vi "AG Spreadsheet.vi"() -> ()   [LabVIEW 2012]
uses:
  Controls/Spreadsheet_Messege.ctl
  <vilib>/Utility/sysdir.llb/System Directory Type.ctl
  Controls/Spreadsheet Commands.ctl
  Utilities/AG Tab Action.ctl
  Controls/Sheet Colors.ctl
  ActivityGuideEvents.ctl
panel:
  in  "Clear Sheet":bool
  in  "Copy to Clipboard":bool
  in  "Save as .csv":bool
  in  "Blank Button":bool
  in  "Sheet Colors":T1={"Header Color"=16711680, "Header Font Color"=16448250, "Font Color"=0, "Clear Color"=16448250, "Alt Clear Color"=13224393}
  in  "Resources":path[](array[path])
  in  "TabButtonsRef":refnum<vi>
  in  "Multicolumn Listbox":i32[](listbox)
  in  "ActivityGuideEvents":T2
  # "Spreadsheet Title"
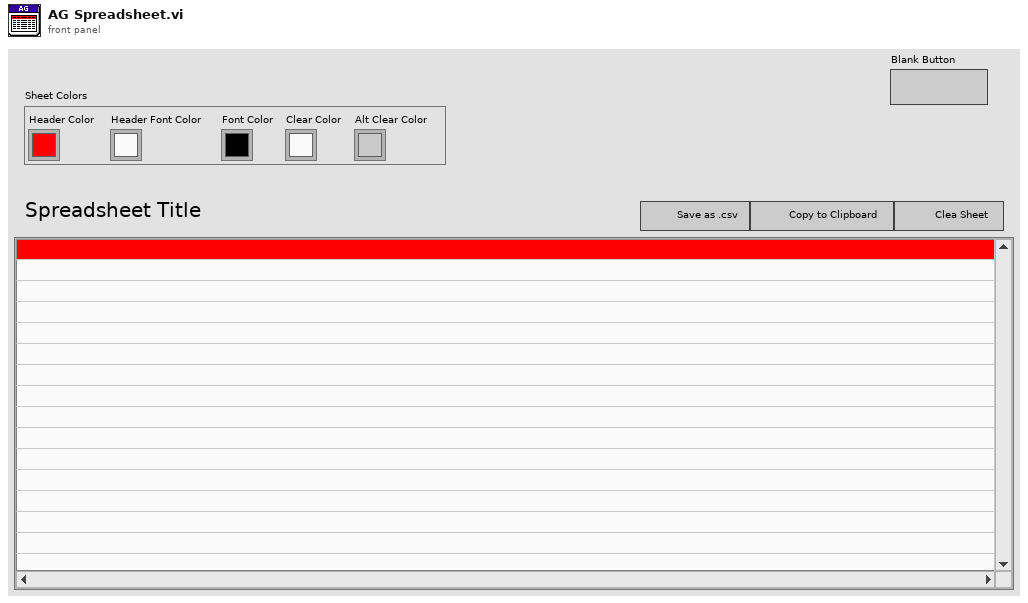
[diagram p1: front panel]
types:
  T1 = typedef "Sheet Colors.ctl" = cluster{"Header Color":u32, "Header Font Color":u32, "Font Color":u32, "Clear Color":u32, "Alt Clear Color":u32}
  T2 = typedef "ActivityGuideEvents.ctl" = refnum<event-registration>
  T3 = typedef "AG Tab Action.ctl" = enum16{"Initilize", "Select", "Blink", "Disable", "KeyFocus", "Set Description", "Hide", "NULL"}
  T4 = typedef "Spreadsheet Commands.ctl" = enum16{"Init", "Clear", "Add", "Mass Add", "Delete Row", "Format Colors"}
  T5 = typedef "Spreadsheet_Messege.ctl" = cluster{"Action (add)":T4, "Data":string[], "2D Data":string[][]}
  T6 = typedef "System Directory Type.ctl" = i32
  T7 = typedef "LVPoint32TypeDef.ctl" = cluster{"Horizontal":i32, "Vertical":i32}
  T8 = typedef "LVRowAndColumnTypeDef.ctl" = cluster{"Row":i32, "Column":i32}
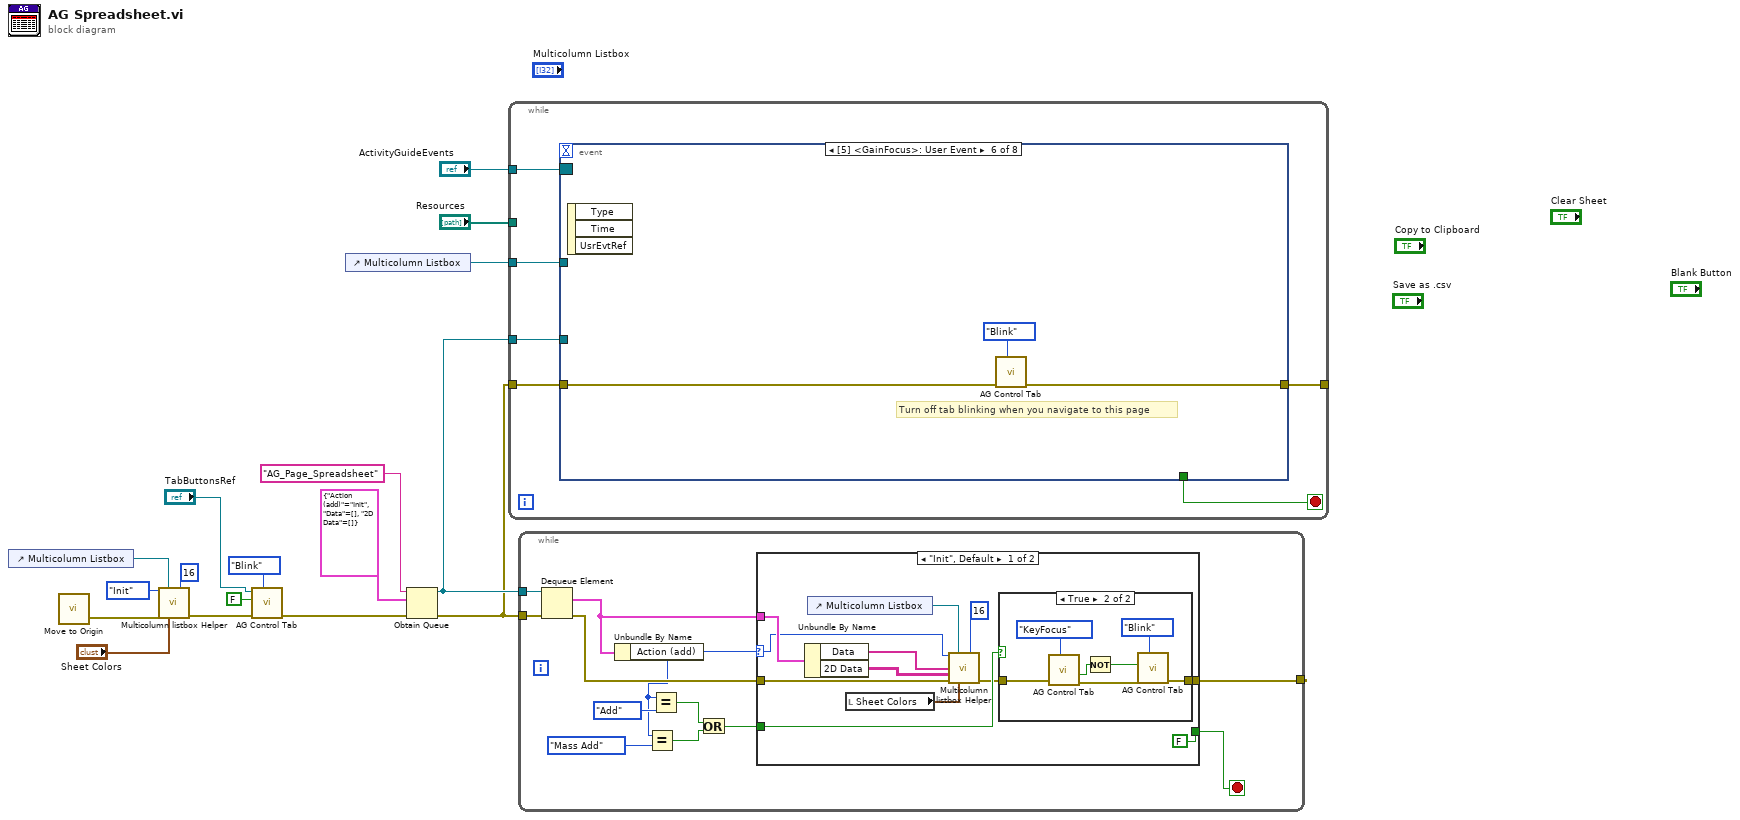
[diagram p0: block diagram]
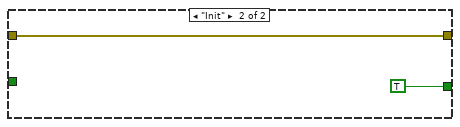
[diagram p3: hidden frame]
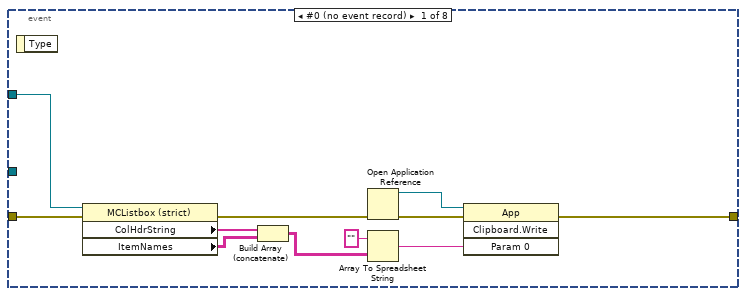
[diagram p4: hidden frame]
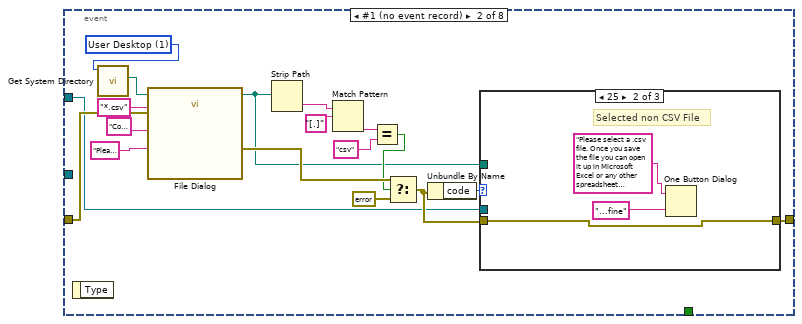
[diagram p5: hidden frame]
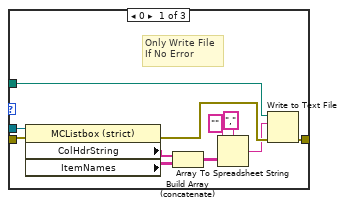
[diagram p6: hidden frame]
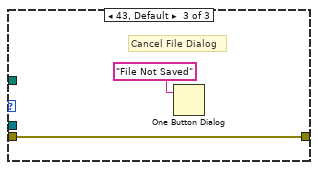
[diagram p7: hidden frame]
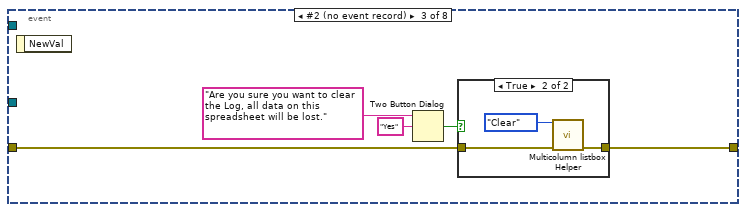
[diagram p8: hidden frame]
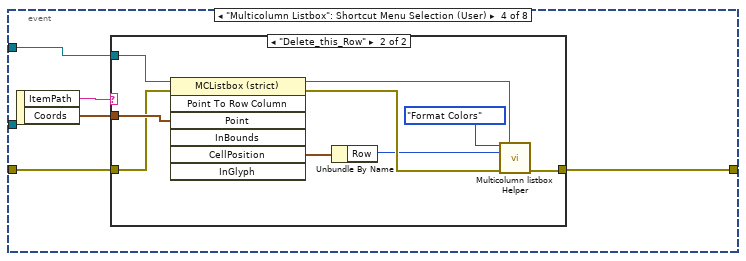
[diagram p10: hidden frame]
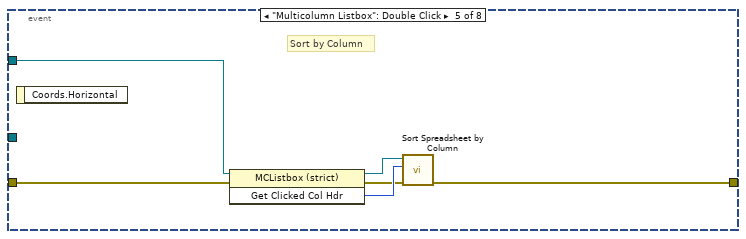
[diagram p12: hidden frame]
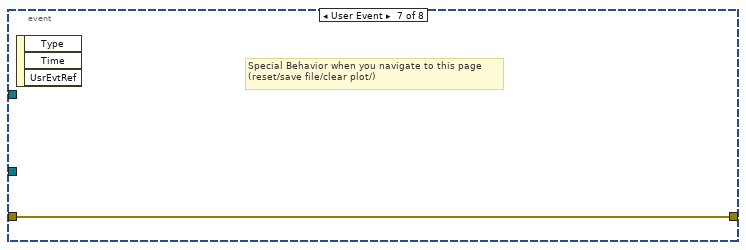
[diagram p13: hidden frame]
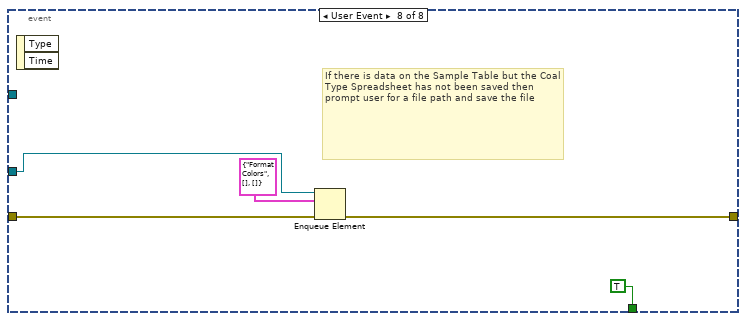
[diagram p14: hidden frame]
diagram:
  n1 = control-ref of="Multicolumn Listbox"() -> (w11:refnum<vi>)
  n2 = call "Move to Origin.vi"() -> ("Error Out"=w2:errorcluster)  [unwired: 3 in]
  n3 = call "Multicolumn listbox Helper.vi"("Action (add default)"=Spreadsheet_Commands."Init", "Multicolumn Ref"=w11, "Visible rows"=16, "Error In"=w2, "Sheet Colors"="Sheet Colors") -> ("Error Out"=w7:errorcluster)  [unwired: 10 in]
  n4 = call "AG Control Tab.vi"("Action (Init)"=AG_Tab_Action."Blink" ("Action"), "error in (no error)"=w7, "Value(F)"=FALSE, "TabButtonsRef"="TabButtonsRef") -> ("error out"=w1:errorcluster)  [unwired: 4 in, 3 out]
  n5 = control-ref of="Multicolumn Listbox"() -> (w13:refnum<vi>)
  n6 = Obtain Queue(name (unnamed)="AG_Page_Spreadsheet", element data type=T5 {"Action (add)"=enum."Init", "Data"=[], "2D Data"=[]} ("Cluster"), error in (no error)=w1) -> (queue out=w14:refnum<queue>, error out=w10:errorcluster)  [unwired: 2 in, 1 out]
  n7 = while {
    tunnel: "ActivityGuideEvents" -> [w23]
    tunnel: w14 -> [w21]
    tunnel: w13 -> [w20]
    tunnel: [w19] -> _
    tunnel: w10 -> [w18]
    tunnel: "Resources" -> [_]
    stop <- w22 stop-if-true
    n8 = event shown="[5] <GainFocus>: User Event" {
      selector: w23 -> [_ _ _ _ _ _ _ _]
      dyn-events: _ -> [_ _ _ _ _ _ _ _]
      timeout: _ -> [_ _ _ _ _ _ _ _]
      tunnel: [_ _ _ _ _ _ _ TRUE] -> w22
      tunnel: w21 -> [_ _ _ _ _ _ _ w103]
      tunnel: w20 -> [w31 w35 _ w78 w95 _ _ _]
      tunnel: [w27 w38 w70 w81 w94 w100 w102 w105] -> w19
      tunnel: w18 -> [w25 w36 w69 w80 w93 w99 w102 w104]
      event #0 (no event record) {
        n9 = event-data() -> ()  [unwired: 1 in, 1 out]
        n10 = property class="MCListbox (strict)"(reference=w31, error in=w25) -> (error out=w26:errorcluster, "ColHdrString"=w30:string[], "ItemNames"=w29:string[][])  [unwired: 1 out]
        n11 = Build Array (concatenate)(w30, w29) -> (w28:string[][])
        n12 = Open Application Reference(8:w26) -> (0:w32:errorcluster, 3:w24:refnum<vi>)  [unwired: 3 in]
        n13 = Array To Spreadsheet String(array=w28, 3:"" ("format string")) -> (spreadsheet string=w33:string)  [unwired: 1 in]
        n14 = invoke class="App" method="Clipboard.Write"(reference=w24, error in=w32, "Param 0"=w33) -> (error out=w27:errorcluster)  [unwired: 1 in, 3 out]
      }
      event #1 (no event record) {
        w50 = T6 1 items=["User Home"=0, "User Desktop"=1, "User Documents"=2, "User Application Data"=3, "User Preferences"=4, "User Temporary"=5, "Public Documents"=6, "Public Application Data"=7, "Public Preferences"=8, "Public Cache"=13, "System Core Libraries"=9, "System Installed Libraries"=10, "Application Files"=11, "Boot Volume Root"=12] ("system directory type")
        n15 = event-data() -> ()  [unwired: 1 in, 1 out]
        n16 = call <vilib>:"Get System Directory.vi"("system directory type"=w50) -> ("system directory"=w49:path)  [unwired: 10 in]
        n17 = call "File Dialog"("start path"=w49, "prompt"="Please select a file to save your data.", "error in"=w36, "pattern (all files)"="*.csv", "pattern label"="Comma Seperated Value Files") -> ("selected path"=w39:path, "error out"=w42:errorcluster)  [unwired: 7 in, 2 out]
        n18 = Strip Path(path=w39) -> (name=w46:string)  [unwired: 1 out]
        n19 = Match Pattern(string=w46, regular expression="[.]") -> (after substring=w45:string)  [unwired: 1 in, 3 out]
        n20 = Equal?(x=w45, y="csv") -> (x = y?=w40:bool)
        n21 = Select(t=w42, s=w40, f=errorcluster {"status"=TRUE, "code"=25, "source"=""}) -> (s? t:f=w37:errorcluster)
        n22 = Unbundle By Name(w37) -> ("code"=w43:i32)
        n23 = case shown="25" w43 {
          tunnel: w39 -> [w63 _ _]
          tunnel: [w62 w64 w67] -> w38
          tunnel: w37 -> [w55 w64 w67]
          tunnel: w35 -> [w54 _ _]
          frame 0 {
            # "Only Write File\nIf No Error"
            n24 = property class="MCListbox (strict)"(reference=w54, error in=w55) -> (error out=w56:errorcluster, "ColHdrString"=w57:string[], "ItemNames"=w58:string[][])  [unwired: 1 out]
            n25 = Build Array (concatenate)(w57, w58) -> (w59:string[][])
            n26 = Array To Spreadsheet String(delimiter (Tab)=",", array=w59, 3:"" ("format string")) -> (spreadsheet string=w53:string)
            n27 = Write to Text File(file (use dialog)=w63, text=w53, error in=w56) -> (error out=w62:errorcluster)  [unwired: 1 in, 2 out]
          }
          frame 25 {
            # "Selected non CSV File"
            n28 = One Button Dialog(message="Please select a .csv file. Once you save the file you can open it up in Microsoft Excel or any other spreadsheet application. ", button name ("OK")="...fine" ("format string")) -> ()  [unwired: 1 out]
          }
          frame 43, Default {
            # "Cancel File Dialog"
            n29 = One Button Dialog(message="File Not Saved") -> ()  [unwired: 1 in, 1 out]
          }
        }
      }
      event #2 (no event record) {
        n30 = event-data() -> ()  [unwired: 1 in, 1 out]
        n31 = Two Button Dialog(message="Are you sure you want to clear the Log, all data on this spreadsheet will be lost.", 2:"Yes" ("T button name (\"OK\")")) -> (T button?=w71:bool)  [unwired: 1 in]
        n32 = case shown="True" w71 {
          tunnel: [w74 w77] -> w70
          tunnel: w69 -> [w74 w76]
          frame False {
          }
          frame True {
            n33 = call "Multicolumn listbox Helper.vi"("Action (add default)"=Spreadsheet_Commands."Clear", "Error In"=w76) -> ("Error Out"=w77:errorcluster)  [unwired: 13 in]
          }
        }
      }
      event "Multicolumn Listbox": Shortcut Menu Selection (User) {
        n34 = event-data() -> ("ItemPath"=w82:string, "Coords"=w79:T7)  [unwired: 1 in]
        n35 = case shown="\"Delete_this_Row\"" w82 {
          tunnel: [w83 w87] -> w81
          tunnel: w80 -> [w83 w90]
          tunnel: w79 -> [_ w92]
          tunnel: w78 -> [_ w84]
          frame "NULL", Default {
          }
          frame "Delete_this_Row" {
            n36 = invoke class="MCListbox (strict)" method="Point To Row Column"(reference=w84, error in=w90, "Point"=w92) -> (reference out=w89:refnum<vi>, error out=w88:errorcluster, "CellPosition"=w91:T8)  [unwired: 4 in, 4 out]
            n37 = Unbundle By Name(w91) -> ("Row"=w85:i32)
            n38 = call "Multicolumn listbox Helper.vi"("Action (add default)"=Spreadsheet_Commands."Format Colors", "Multicolumn Ref"=w89, "Row to Delete"=w85, "Error In"=w88) -> ("Error Out"=w87:errorcluster)  [unwired: 11 in]
          }
        }
      }
      event "Multicolumn Listbox": Double Click {
        # "Sort by Column"
        n39 = event-data() -> ()  [unwired: 1 in, 1 out]
        n40 = invoke class="MCListbox (strict)" method="Get Clicked Col Hdr"(reference=w95, error in=w93) -> (reference out=w97:refnum<vi>, error out=w96:errorcluster, "Get Clicked Column Header"=w98:i32)  [unwired: 1 in]
        n41 = call "Sort Spreadsheet by Column.vi"("error in (no error)"=w96, "Column Number"=w98, "Ref In"=w97) -> ("error out"=w94:errorcluster)  [unwired: 8 in]
      }
      event User Event {
        # "Turn off tab blinking when you navigate to this page"
        n42 = event-data() -> ()  [unwired: 1 in, 3 out]
        n43 = call "AG Control Tab.vi"("Action (Init)"=AG_Tab_Action."Blink" ("Action"), "error in (no error)"=w99) -> ("error out"=w100:errorcluster)  [unwired: 6 in, 3 out]
      }
      event User Event {
        # "Special Behavior when you navigate to this page\n(reset/save file/clear plot/)"
        n44 = event-data() -> ()  [unwired: 1 in, 3 out]
      }
      event User Event {
        # "If there is data on the Sample Table but the Coal Type Spreadsheet has not been saved then prompt user for a file path and save the file"
        n45 = event-data() -> ()  [unwired: 1 in, 2 out]
        n46 = Enqueue Element(queue=w103, element=T5 {"Action (add)"=enum."Format Colors", "Data"=[], "2D Data"=[]}, error in (no error)=w104) -> (error out=w105:errorcluster)  [unwired: 1 in, 2 out]
      }
    }
  }
  n47 = while {
    tunnel: w14 -> [w119]
    tunnel: w10 -> [w118]
    tunnel: [w108] -> _
    stop <- w117 stop-if-true
    n48 = Dequeue Element(queue=w119, error in (no error)=w118) -> (element=w115:T5, error out=w116:errorcluster)  [unwired: 1 in, 2 out]
    n49 = Unbundle By Name(w115) -> ("Action (add)"=w110:T4)
    n50 = Equal?(x=w110, y=Spreadsheet_Commands."Mass Add" ("Action (add)")) -> (x = y?=w113:bool)
    n51 = Equal?(x=w110, y=Spreadsheet_Commands."Add" ("Action (add)")) -> (x = y?=w114:bool)
    n52 = Or(x=w114, y=w113) -> (x .or. y?=w109:bool)
    n53 = case shown="\"Init\", Default" w110 {
      selector: w110 -> [w125 _]
      tunnel: [FALSE TRUE] -> w117
      tunnel: w116 -> [w130 w140]
      tunnel: w115 -> [w129 _]
      tunnel: w109 -> [w123 _]
      tunnel: [w121 w140] -> w108
      frame "Init", Default {
        n54 = Unbundle By Name(w129) -> ("Data"=w127:string[], "2D Data"=w124:string[][])
        n55 = control-ref of="Multicolumn Listbox"() -> (w126:refnum<vi>)
        n56 = local read "Sheet Colors"() -> (w120:T1)
        n57 = call "Multicolumn listbox Helper.vi"("Action (add default)"=w125, "Multicolumn Ref"=w126, "Visible rows"=16, "Data"=w127, "2D Data"=w124, "Error In"=w130, "Sheet Colors"=w120) -> ("Error Out"=w122:errorcluster)  [unwired: 8 in]
        n58 = case shown="True" w123 {
          tunnel: w122 -> [w132 w138]
          tunnel: [w132 w139] -> w121
          frame False {
          }
          frame True {
            n59 = call "AG Control Tab.vi"("Action (Init)"=AG_Tab_Action."KeyFocus" ("Action"), "error in (no error)"=w138) -> ("error out"=w135:errorcluster, "Selected?"=w134:bool)  [unwired: 6 in, 2 out]
            n60 = Not(x=w134) -> (.not. x?=w133:bool)
            n61 = call "AG Control Tab.vi"("Action (Init)"=AG_Tab_Action."Blink" ("Action"), "error in (no error)"=w135, "Value(F)"=w133) -> ("error out"=w139:errorcluster)  [unwired: 5 in, 3 out]
          }
        }
      }
      frame "Init" {
      }
    }
  }
